vi "Switch status IO.vi"(3 "String input":T1(array[cluster])=[{"result string"="xA1", "result string"="yA7"}, {"result string"="comD7", "result string"="chD7"}, {"result string"="comC1", "result string"="chC1"}], 5 "Write: T\nRead: F":bool, 6 "Path":path=path "C:/LabView/PPMS basic VIs/Pickering_Switch_Memory.txt") -> (1 "String out":string[](array[string])=["xA1", "yA7", "comD7", "chD7", "comC1", "chC1", ""])   [LabVIEW 2013]
uses:
  PPMS_remote/branches/sim-JL/Simulate.glb.vi
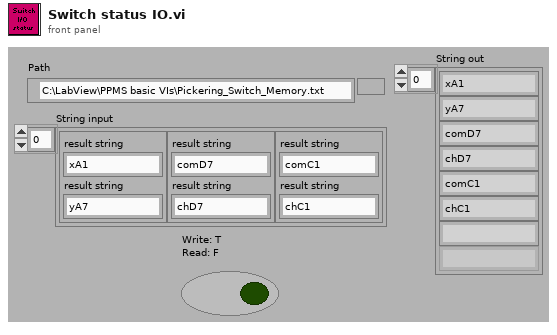
[diagram p1: front panel]
types:
  T1 = cluster{"result string":string, "result string":string}[]
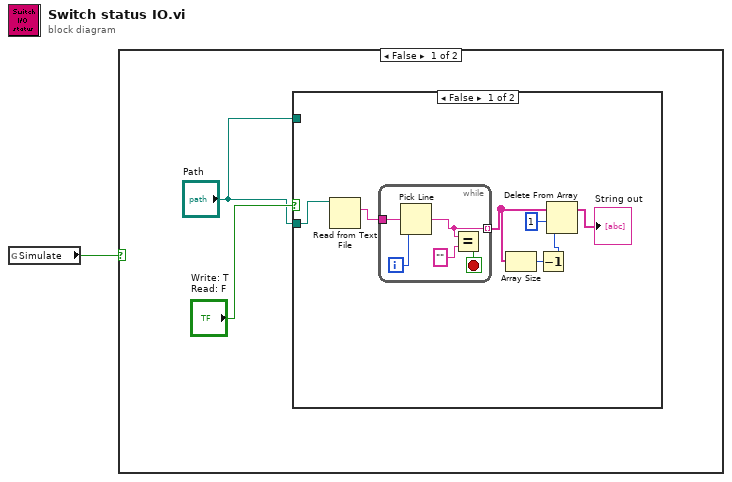
[diagram p0: block diagram]
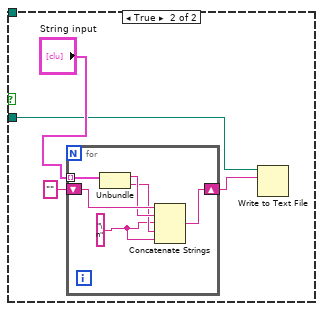
[diagram p2: hidden frame]
diagram:
  n1 = global read "Simulate.glb.vi" "Simulate"() -> (w1:bool)
  n2 = case shown="False" w1 {
    frame False {
      n3 = case shown="False" "Write: T\nRead: F" {
        tunnel: "Path" -> [w9 w17]
        tunnel: "Path" -> [_ _]
        frame False {
          n4 = Read from Text File(file (use dialog)=w9) -> (text=w10:string)  [unwired: 3 in, 3 out]
          n5 = while {
            tunnel: w10 -> [w15]
            tunnel: [w13] -> w8 mode=indexing
            i -> [w14]
            stop <- w11 stop-if-true
            n6 = Pick Line(multi-line string=w15, line index=w14) -> (output string=w13:string)  [unwired: 1 in]
            n7 = Equal?(x=w13, y="" ("output string")) -> (x = y?=w11:bool)
          }
          n8 = Array Size(array=w8) -> (size(s)=w7:i32)
          n9 = Decrement(x=w7) -> (x-1=w6:i32)
          n10 = Delete From Array(array=w8, length=1, index=w6) -> (array with subset deleted=→"String out":string[])  [unwired: 1 out]
        }
        frame True {
          n11 = for {
            tunnel: "String input" -> [w25] mode=indexing
            shift-right: [w24] -> w16
            shift-left: "" -> [w23]
            w20 = "\n"
            n12 = Unbundle(w25) -> ("result string"=w22:string, "result string"=w21:string)
            n13 = Concatenate Strings(w23, w22, w20, w21, w20) -> (w24:string)
          }
          n14 = Write to Text File(file (use dialog)=w17, text=w16) -> ()  [unwired: 2 in, 3 out]
        }
      }
    }
    frame True {
    }
  }
